vi "STS_Connect.vi"(8 "error in":errorcluster, 11 "Address Cluster out输入":T1 {"PCU_communcation_method" items=["GPIB", "C232C", "TCPIP", "USB"]; "tsl_communcation_method" items=["GPIB", "C232C", "TCPIP", "USB"]; "MPM_communcation_method" items=["GPIB", "C232C", "TCPIP", "USB"]}) -> (0 "error out":errorcluster, 3 "Address Cluster out":T1 {"PCU_communcation_method" items=["GPIB", "C232C", "TCPIP", "USB"]; "tsl_communcation_method" items=["GPIB", "C232C", "TCPIP", "USB"]; "MPM_communcation_method" items=["GPIB", "C232C", "TCPIP", "USB"]})   [LabVIEW 2017]
uses:
  CTL/Address Cluster.ctl
  D:/test/PDLSTS/LV_PDL_Sample/DLL/InstrumentDLL.dll
  DLL/InstrumentDLL.dll
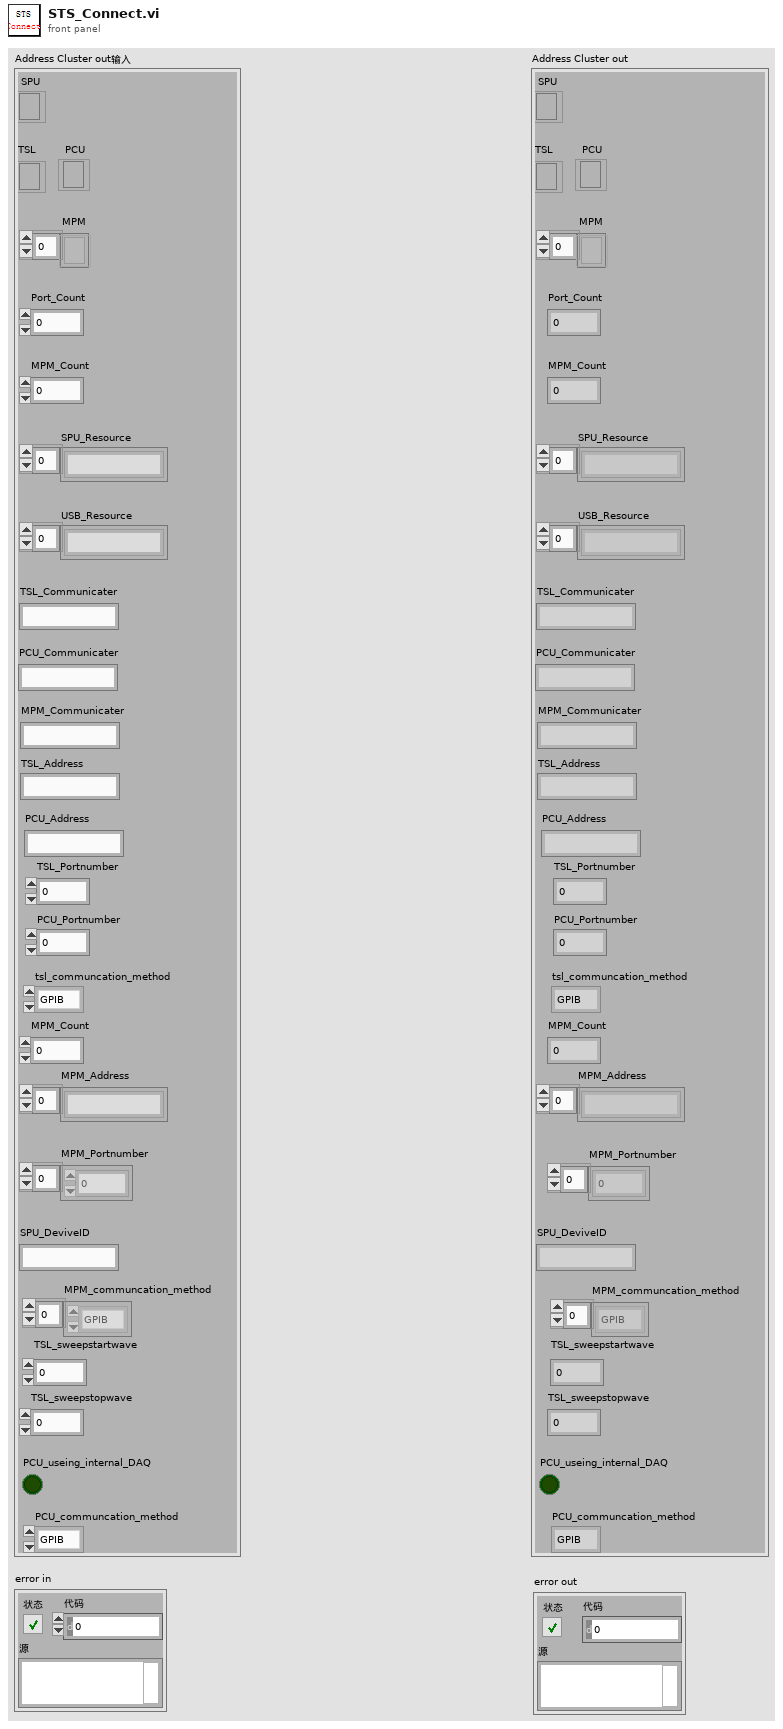
[diagram p1: front panel]
types:
  T1 = typedef "Address Cluster.ctl" = cluster{"SPU":refnum<k24>, "MPM":refnum<k24>[], "Port_Count":dbl, "MPM_Count":dbl, "SPU_Resource":string[], "USB_Resource":string[], "MPM_Communicater":string, "MPM_Count":dbl, "MPM_Address":string[], "MPM_Portnumber":dbl[], "SPU_DeviveID":string, "MPM_communcation_method":i32[], "TSL_sweepstartwave":dbl, "TSL_sweepstopwave":dbl, "TSL_Address":string, "TSL_Communicater":string, "TSL":refnum<k24>, "tsl_communcation_method":i32, "TSL_Portnumber":dbl, "PCU":refnum<k24>, "PCU_Communicater":string, "PCU_Address":string, "PCU_Portnumber":dbl, "PCU_useing_internal_DAQ":bool, "PCU_communcation_method":i32}
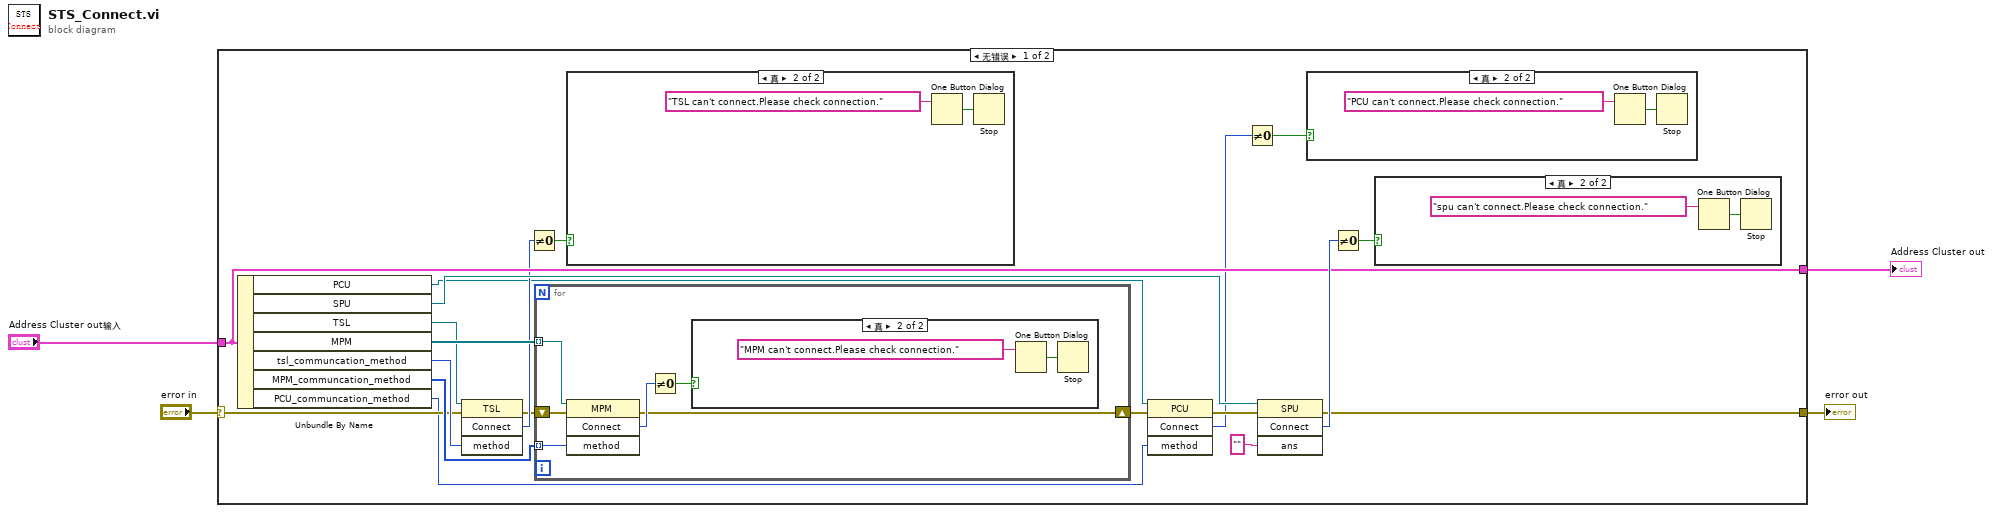
[diagram p0: block diagram]
diagram:
  n1 = case shown="无错误" "error in" {
    selector: "error in" -> [w16 w40]
    tunnel: "Address Cluster out输入" -> [w15 w39]
    tunnel: [w11 w40] -> w2
    tunnel: [w15 w39] -> w1
    frame No Error {
      n2 = Unbundle By Name(w15) -> ("PCU"=w10:refnum<k24>, "SPU"=w22:refnum<k24>, "TSL"=w18:refnum<k24>, "MPM"=w20:refnum<k24>[], "tsl_communcation_method"=w19:i32, "MPM_communcation_method"=w21:i32[], "PCU_communcation_method"=w9:i32)
      n3 = invoke on="调用节点" class="TSL" method="Connect"(reference=w18, error in=w16, "method"=w19) -> (error out=w12:errorcluster, "Connect"=w14:i32)  [unwired: 1 in, 2 out]
      n4 = Not Equal To 0?(x=w14) -> (x != 0?=w13:bool)
      n5 = for {
        tunnel: w20 -> [w36] mode=indexing
        tunnel: w21 -> [w35] mode=indexing
        shift-right: [w32] -> w8
        shift-left: w12 -> [w31]
        n6 = invoke on="调用节点" class="MPM" method="Connect"(reference=w36, error in=w31, "method"=w35) -> (error out=w32:errorcluster, "Connect"=w33:i32)  [unwired: 1 in, 2 out]
        n7 = Not Equal To 0?(x=w33) -> (x != 0?=w34:bool)
        n8 = case shown="真" w34 {
          frame False {
          }
          frame True {
            n9 = One Button Dialog(message="MPM can't connect.Please check connection." ("消息")) -> (true=w37:bool)  [unwired: 1 in]
            n10 = Stop(stop? (T)=w37) -> ()
          }
        }
      }
      n11 = case shown="真" w13 {
        frame False {
        }
        frame True {
          n12 = One Button Dialog(message="TSL can't connect.Please check connection." ("消息")) -> (true=w27:bool)  [unwired: 1 in]
          n13 = Stop(stop? (T)=w27) -> ()
        }
      }
      n14 = invoke on="调用节点" class="PCU" method="Connect"(reference=w10, error in=w8, "method"=w9) -> (error out=w7:errorcluster, "Connect"=w6:i32)  [unwired: 1 in, 2 out]
      n15 = Not Equal To 0?(x=w6) -> (x != 0?=w5:bool)
      n16 = invoke class="SPU" method="Connect"(reference=w22, error in=w7, "ans"="") -> (error out=w11:errorcluster, "Connect"=w24:i32)  [unwired: 1 in, 2 out]
      n17 = case shown="真" w5 {
        frame False {
        }
        frame True {
          n18 = One Button Dialog(message="PCU can't connect.Please check connection." ("消息")) -> (true=w25:bool)  [unwired: 1 in]
          n19 = Stop(stop? (T)=w25) -> ()
        }
      }
      n20 = Not Equal To 0?(x=w24) -> (x != 0?=w23:bool)
      n21 = case shown="真" w23 {
        frame False {
        }
        frame True {
          n22 = One Button Dialog(message="spu can't connect.Please check connection." ("消息")) -> (true=w29:bool)  [unwired: 1 in]
          n23 = Stop(stop? (T)=w29) -> ()
        }
      }
    }
    frame Error {
    }
  }
  "Address Cluster out" <- w1
  "error out" <- w2
